vi "SaveStriptestRecoveryFiles.vi"(2 "Arrays format":string, 3 "Array Titles":string, 4 "Strip Segment":string, 5 "no. of arrays":i32, 6 "Actual array lengths":i32, 7 "Region #":u32) -> (0 "Path + Filename OUT":string, 1 "Filename OUT":string)   [LabVIEW 2018]
uses:
  general_VIs/globals/QC_RunInformation.vi
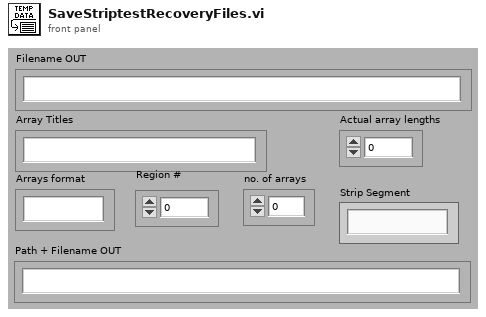
[diagram p1: front panel]
types:
  T1 = enum16{"open", "open or create", "create or replace", "create"}
  T2 = cluster{"Institute":string, "Manufacturers":string[], "Devices":string[], "Serialnumbers Lookup DB":string, "Data directory":string, "Backup & screenshot directory":string, "List of known users":string[]}
  T3 = enum16{"Reset", "Read Array", "Read Element", "Write Element", "Write Array", "Add Element", "Add Array"}
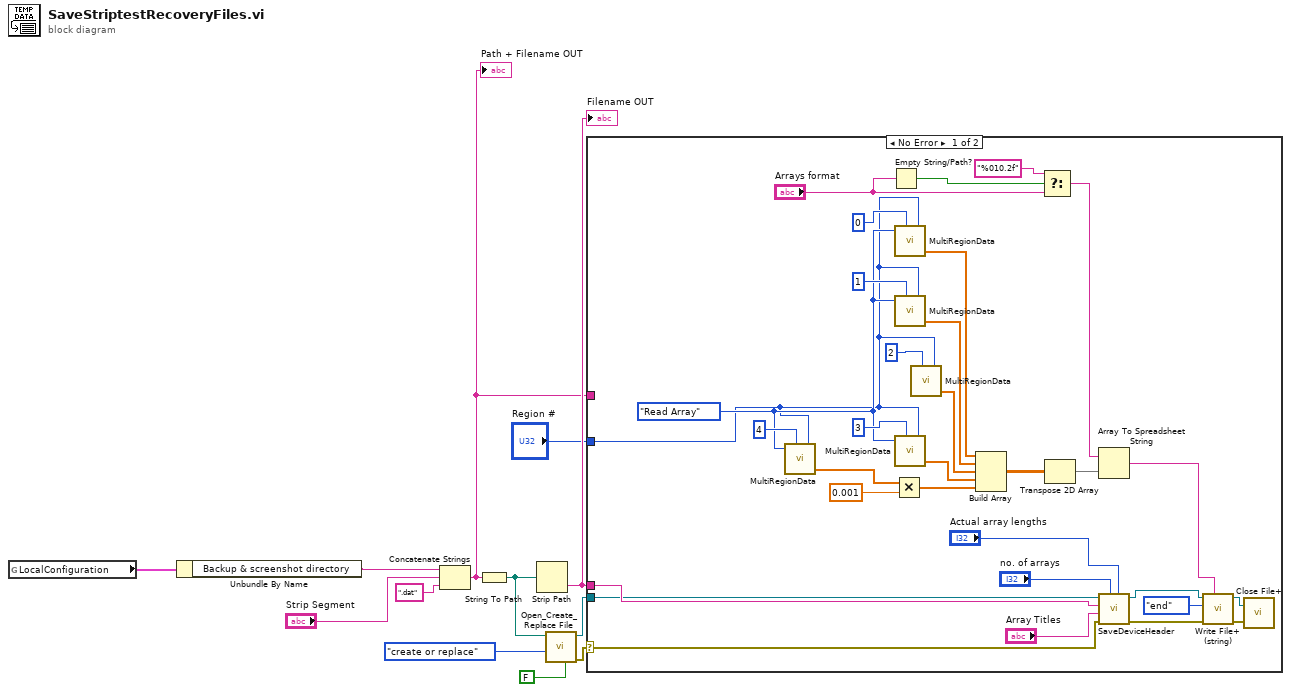
[diagram p0: block diagram]
diagram:
  n1 = global read "QC_RunInformation.vi" "LocalConfiguration"() -> (w4:T2)
  n2 = Unbundle By Name(w4) -> ("Backup & screenshot directory"=w3:string)
  n3 = Concatenate Strings(w3, "Strip Segment", ".dat") -> (w6:string)
  "Path + Filename OUT" <- w6
  n4 = String To Path(string=w6) -> (path=w9:path)
  n5 = Strip Path(path=w9) -> (name=w10:string)  [unwired: 1 out]
  "Filename OUT" <- w10
  n6 = call <vilib>:"Open_Create_Replace File.vi"("advisory dialog? (display:T)"=FALSE, "function (open:0)"=T1."create or replace", "file path"=w9) -> ("error out"=w8:errorcluster, "refnum"=w11:refnum<file>)  [unwired: 5 in, 2 out]
  n7 = case shown="No Error" w8 {
    selector: w8 -> [w44 _]
    tunnel: w11 -> [w41 _]
    tunnel: w6 -> [_ _]
    tunnel: w10 -> [w42 _]
    tunnel: "Region #" -> [w17 _]
    frame No Error {
      w26 = T3."Read Array" ("Action")
      n8 = call "MultiRegionData.vi"("Action"=w26, "Array No."=4, "Region index"=w17) -> ("Array OUT"=w24:dbl[])  [unwired: 3 in, 1 out]
      n9 = Empty String/Path?(string/path="Arrays format") -> (empty?=w38:bool)
      n10 = Multiply(x=w24, y=0.001) -> (x*y=w23:dbl[])
      n11 = call "MultiRegionData.vi"("Action"=w26, "Array No."=0, "Region index"=w17) -> ("Array OUT"=w19:dbl[])  [unwired: 3 in, 1 out]
      n12 = call "MultiRegionData.vi"("Action"=w26, "Array No."=1, "Region index"=w17) -> ("Array OUT"=w20:dbl[])  [unwired: 3 in, 1 out]
      n13 = call "MultiRegionData.vi"("Action"=w26, "Array No."=3, "Region index"=w17) -> ("Array OUT"=w22:dbl[])  [unwired: 3 in, 1 out]
      n14 = call "MultiRegionData.vi"("Array No."=2, "Region index"=w17) -> ("Array OUT"=w21:dbl[])  [unwired: 4 in, 1 out]
      n15 = Build Array(w19, w20, w21, w22, w23) -> (w18:dbl[][])
      n16 = Select(t="%010.2f", s=w38, f="Arrays format") -> (s? t:f=w32:string)
      n17 = Transpose 2D Array(2D array=w18) -> (transposed array=w16:dbl[][])
      n18 = Array To Spreadsheet String(array=w16, 3:w32) -> (spreadsheet string=w15:string)  [unwired: 1 in]
      n19 = call "SaveDeviceHeader.vi"("Array Lengths"="Actual array lengths", "no. of arrays"="no. of arrays", "error in (no error)"=w44, "Array Titles"="Array Titles", "Filename"=w42, "File Refnum in"=w41) -> ("error out"=w13:errorcluster, "File Refnum out"=w14:refnum<file>)  [unwired: 3 in, 1 out]
      n20 = call <vilib>:"Write File+ (string).vi"("string"=w15, "error in (no error)"=w13, "pos mode (rel. to end:1)"=enum16{"start", "end", "current"}."end", "refnum"=w14) -> ("error out"=w34:errorcluster, "dup refnum"=w35:refnum<file>)  [unwired: 3 in, 1 out]
      n21 = call <vilib>:"Close File+.vi"("error in (no error)"=w34, "refnum"=w35) -> ()  [unwired: 3 in, 3 out]
    }
    frame Error {
    }
  }
